vi "GPSmain.vi"() -> ()   [LabVIEW 2010]
uses:
  _types/FixQuality.ctl
  _typedefs/GPS Coordinate.ctl
  <vilib>/Instr/_visa.llb/VISA Configure Serial Port (Instr).vi
panel:
  in  "stop 2":bool
  out "concatenated string":string
  in  "COM Port":refnum<visa-resource-name>
  out "Current String":string
  out "XY Graph":cluster{"Y":dbl[], "Y":dbl[]}[](graph)
  out "Read PreError":i32
  out "Configure Iterate Count":i32
  out "Parse Iterate Count":i32
  out "Read Iterate Count":i32
  out "serial Configure Error":errorcluster
  out "Internal Error Read":errorcluster
  out "HDOP":dbl
  out "nSatellites":i32
  out "Time":string
  out "Location":T1 {"Elev. (m)" format="%_12g"; "Lon (deg)" format="%_12g"; "Lat (deg)" format="%_12g"}
  out "2D3D_Automatic?":bool
  out "Valid GPS Fix?":bool
  out "Fix Quality":T2
  out "error out":errorcluster
  in  "stop":bool
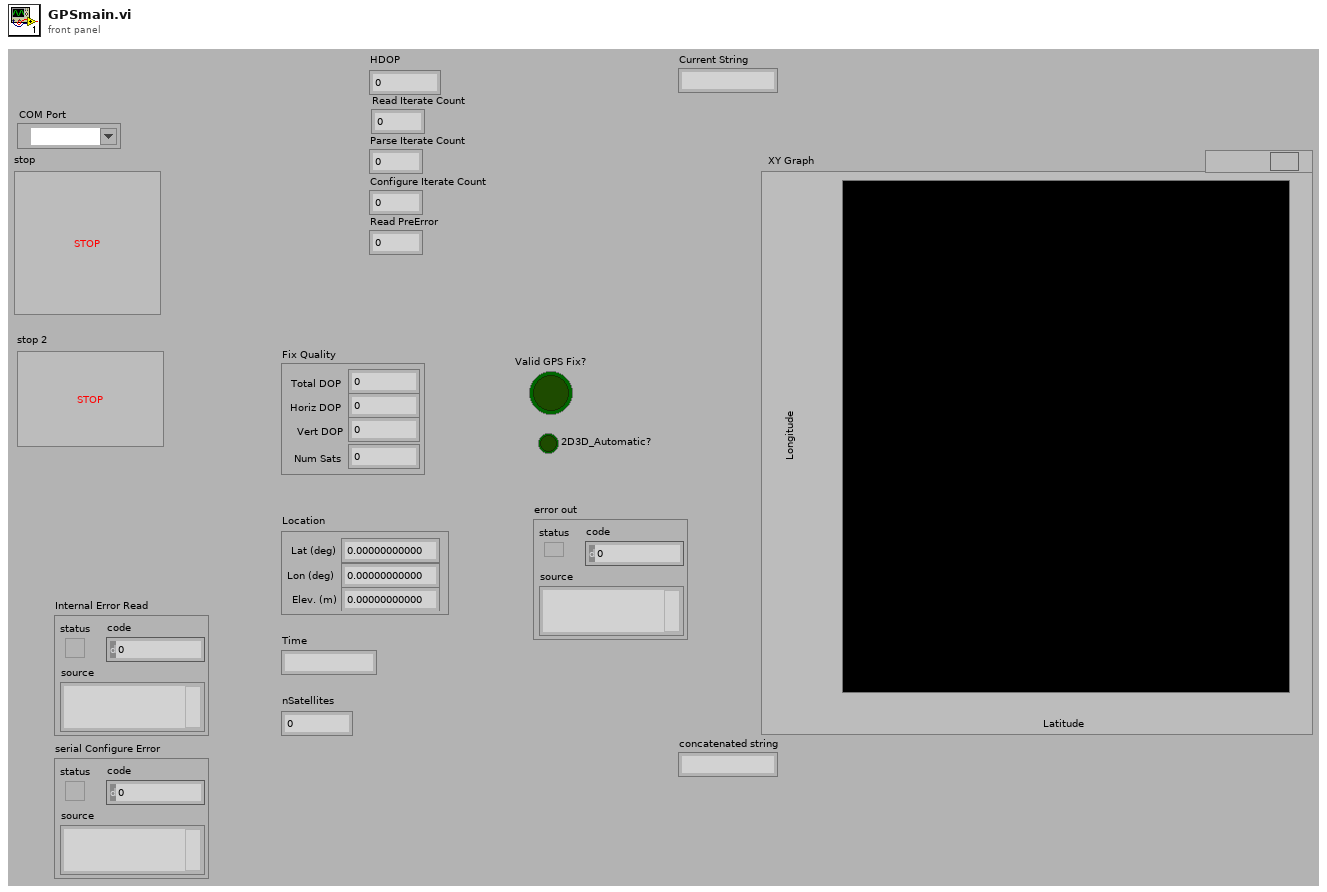
[diagram p1: front panel]
types:
  T1 = typedef "GPS Coordinate.ctl" = cluster{"Lat (deg)":dbl, "Lon (deg)":dbl, "Elev. (m)":dbl}
  T2 = typedef "FixQuality.ctl" = cluster{"Horiz DOP":dbl, "Vert DOP":dbl, "Total DOP":dbl, "Num Sats":i32}
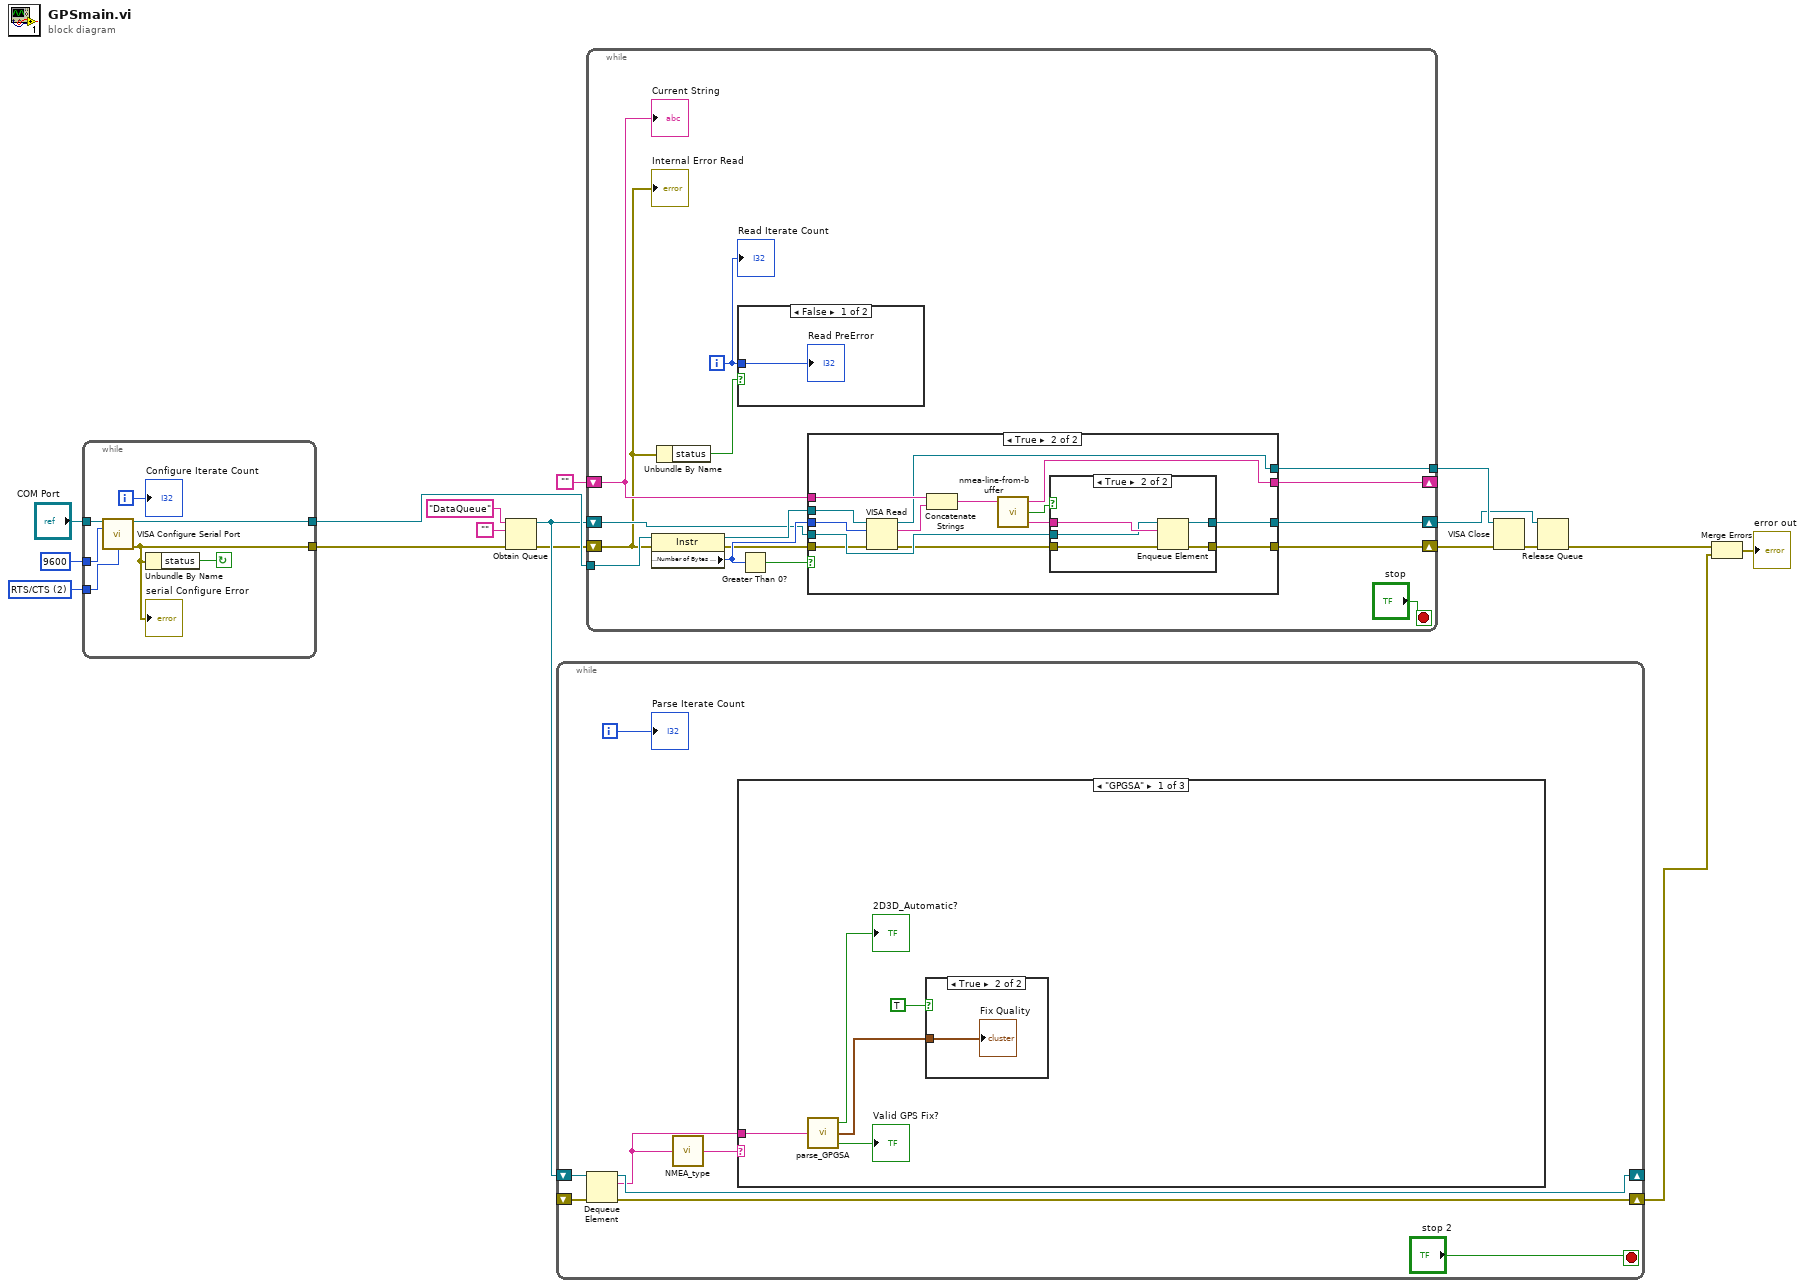
[diagram p0: block diagram]
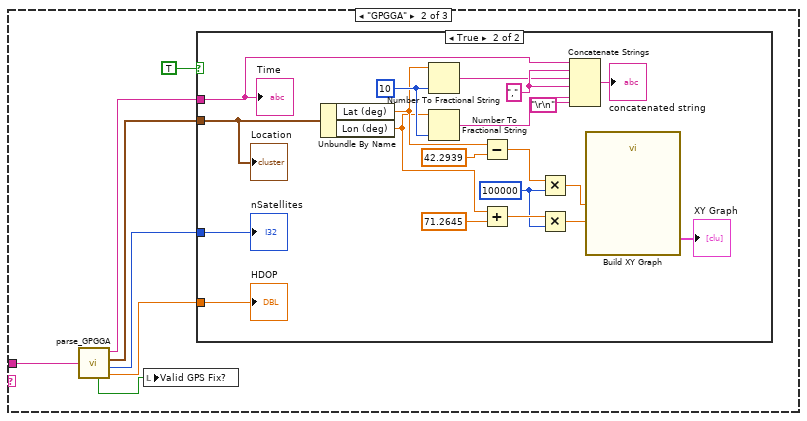
[diagram p3: hidden frame]
diagram:
  w16 = u16 2 items=["None", "XON/XOFF", "RTS/CTS", "XON/XOFF & RTS/CTS", "DTR/DSR", "XON/XOFF & DTR/DSR"] ("flow control (0:none)")
  n1 = while {
    tunnel: 9600 -> [w24]
    tunnel: "COM Port" -> [w23]
    tunnel: w16 -> [w22]
    tunnel: [w20] -> w15
    tunnel: [w19] -> w8
    i -> [w18]
    stop <- w21 continue-if-true
    n2 = call-poly "VISA Configure Serial Port"("VISA resource name"=w23, "baud rate (9600)"=w24, "flow control (0:none)"=w22) -> ("VISA resource name out"=w20:refnum<visa-resource-name>, "error out"=w19:errorcluster)  [unwired: 11 in]
    "serial Configure Error" <- w19
    n3 = Unbundle By Name(w19) -> ("status"=w21:bool)
    "Configure Iterate Count" <- w18
  }
  n4 = Obtain Queue(name (unnamed)="DataQueue", element data type="", error in (no error)=w8) -> (queue out=w9:refnum<queue>, error out=w7:errorcluster)  [unwired: 2 in, 1 out]
  n5 = while {
    shift-right: [w31] -> _
    shift-left: w9 -> [w32]
    shift-right: [w27] -> w1
    shift-left: _ -> [w28]
    i -> [w26]
    stop <- "stop 2" stop-if-true
    n6 = Dequeue Element(queue=w32, error in (no error)=w28) -> (queue out=w31:refnum<queue>, element=w29:string, error out=w27:errorcluster)  [unwired: 1 in, 1 out]
    n7 = call "NMEA_type.vi"("NMEA String"=w29) -> ("NMEA Sentence Type"=w30:string)
    n8 = case shown="\"GPGSA\"" w30 {
      tunnel: w29 -> [w37 w45 _]
      frame "GPGSA" {
        n9 = call "parse_GPGSA.vi"("NMEA GPGSA String"=w37) -> ("2D3D_Automatic?"=→"2D3D_Automatic?":bool, "New Fix Quality"=w36:T2, "Valid GPS Fix?"=→"Valid GPS Fix?":bool)
        n10 = case shown="True" TRUE {
          tunnel: w36 -> [_ w38]
          frame False {
          }
          frame True {
            "Fix Quality" <- w38
          }
        }
      }
      frame "GPGGA" {
        n11 = call "parse_GPGGA.vi"("NMEA GPGGA String"=w45) -> ("Valid GPS Fix?"=w40:bool, "Time"=w43:string, "GPS Coordinate"=w44:T1, "nSatellites"=w42:i32, "HDOP"=w41:dbl)  [unwired: 1 in]
        n12 = local write "Valid GPS Fix?"(w40) -> ()
        n13 = case shown="True" TRUE {
          tunnel: w44 -> [_ w63]
          tunnel: w43 -> [_ w53]
          tunnel: w42 -> [_ w65]
          tunnel: w41 -> [_ w64]
          frame False {
          }
          frame True {
            w48 = i16 10 ("width (-)")
            w52 = "," ("string")
            w57 = 100000
            n14 = Unbundle By Name(w63) -> ("Lat (deg)"=w47:dbl, "Lon (deg)"=w46:dbl)
            n15 = Number To Fractional String(number=w47, precision (6)=w48) -> (F-format string=w50:string)  [unwired: 2 in]
            n16 = Number To Fractional String(number=w46, precision (6)=w48) -> (F-format string=w49:string)  [unwired: 2 in]
            n17 = Subtract(x=w47, y=42.2939) -> (x-y=w58:dbl)
            n18 = Add(x=w46, y=71.2645) -> (x+y=w59:dbl)
            n19 = Multiply(x=w58, y=w57) -> (x*y=w56:dbl)
            n20 = Multiply(x=w59, y=w57) -> (x*y=w55:dbl)
            n21 = Concatenate Strings(w53, w52, w50, w52, w49, "\r\n") -> (→"concatenated string":string)
            n22 = call "Build XY Graph"("Y Input"=w55, "X Input"=w56) -> ("XY Graph"=→"XY Graph":cluster{"Y":dbl[], "Y":dbl[]}[])  [unwired: 3 in, 6 out]
            "Location" <- w63
            "Time" <- w53
            "nSatellites" <- w65
            "HDOP" <- w64
          }
        }
      }
      frame Default {
      }
    }
    "Parse Iterate Count" <- w26
  }
  n23 = while {
    tunnel: w15 -> [w80]
    shift-right: [w75] -> _
    shift-left: "" -> [w76]
    shift-right: [w73] -> w10
    shift-left: w9 -> [w74]
    tunnel: [w71] -> w11
    shift-right: [w69] -> w5
    shift-left: w7 -> [w68]
    i -> [w66]
    stop <- "stop" stop-if-true
    n24 = property class="Instr"(reference=w80, error in=w68) -> (reference out=w78:refnum<visa-resource-name>, error out=w70:errorcluster, "Serial Settings:Number of Bytes at Serial Port"=w77:u32)
    n25 = Unbundle By Name(w68) -> ("status"=w67:bool)
    n26 = case shown="False" w67 {
      tunnel: w66 -> [w81 _]
      frame False {
        "Read PreError" <- w81
      }
      frame True {
      }
    }
    n27 = Greater Than 0?(x=w77) -> (x > 0?=w79:bool)
    n28 = case shown="True" w79 {
      tunnel: w78 -> [w83 w99]
      tunnel: w77 -> [_ w98]
      tunnel: w76 -> [w85 w97]
      tunnel: [w85 w94] -> w75
      tunnel: w74 -> [w84 w91]
      tunnel: [w84 w90] -> w73
      tunnel: [w83 w89] -> w71
      tunnel: w70 -> [w82 w88]
      tunnel: [w82 w87] -> w69
      frame False {
      }
      frame True {
        n29 = VISA Read(VISA resource name=w99, byte count=w98, error in (no error)=w88) -> (VISA resource name out=w89:refnum<visa-resource-name>, read buffer=w96:string, error out=w86:errorcluster)  [unwired: 1 out]
        n30 = Concatenate Strings(w97, w96) -> (w95:string)
        n31 = call "nmea-line-from-buffer.vi"("buffer"=w95) -> ("line"=w92:string, "new line?"=w93:bool, "remaining buffer"=w94:string)  [unwired: 2 in]
        n32 = case shown="True" w93 {
          tunnel: w92 -> [_ w106]
          tunnel: w91 -> [w101 w105]
          tunnel: [w101 w104] -> w90
          tunnel: [w100 w103] -> w87
          tunnel: w86 -> [w100 w102]
          frame False {
          }
          frame True {
            n33 = Enqueue Element(queue=w105, element=w106, error in (no error)=w102) -> (queue out=w104:refnum<queue>, error out=w103:errorcluster)  [unwired: 1 in, 1 out]
          }
        }
      }
    }
    "Internal Error Read" <- w68
    "Read Iterate Count" <- w66
    "Current String" <- w76
  }
  n34 = VISA Close(VISA resource name=w11, error in (no error)=w5) -> (error out=w6:errorcluster)
  n35 = Release Queue(queue=w10, error in (no error)=w6) -> (error out=w4:errorcluster)  [unwired: 1 in, 2 out]
  n36 = Merge Errors(w4, w1) -> (→"error out":errorcluster)
